vi "Power.vi"(8 "error in (no error)":errorcluster, 10 "Waveform in":waveform(dbl), 11 "RFID system in":refnum<class "RFID system.lvclass">) -> (0 "error out":errorcluster, 3 "RFID system out":refnum<class "RFID system.lvclass">, 5 "Waveform out":waveform(dbl))   [LabVIEW 2019, in "RFID system.lvclass"]
uses:
  RFID system.lvclass
  <vilib>/measure/madcrms.llb/Averaged DC-RMS for 1 Chan.vi
  <vilib>/measure/NI_MAPro.lvlib
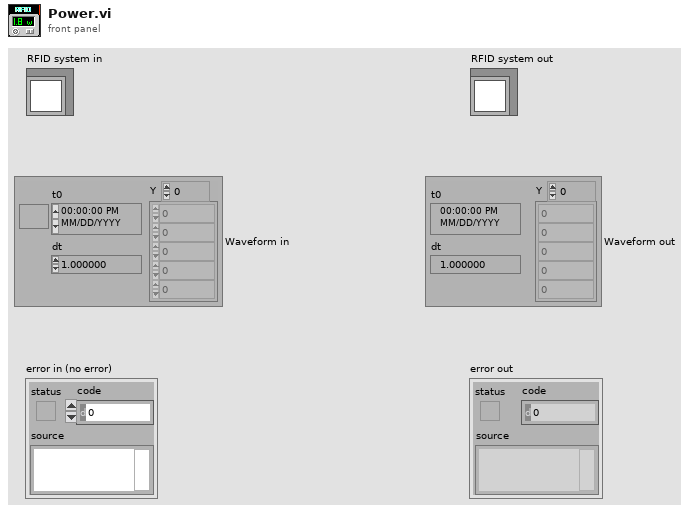
[diagram p1: front panel]
types:
  T1 = cluster{"window for DC":enum16{"Rectangular (none)", "Hanning", "Low side lobe"}, "output function":enum16{"DC only", "RMS only", "DC and RMS"}, "window for RMS":enum16{"Rectangular (none)", "Hanning", "Low side lobe"}, "exp. time constant":dbl, "Ignore input start time":bool}
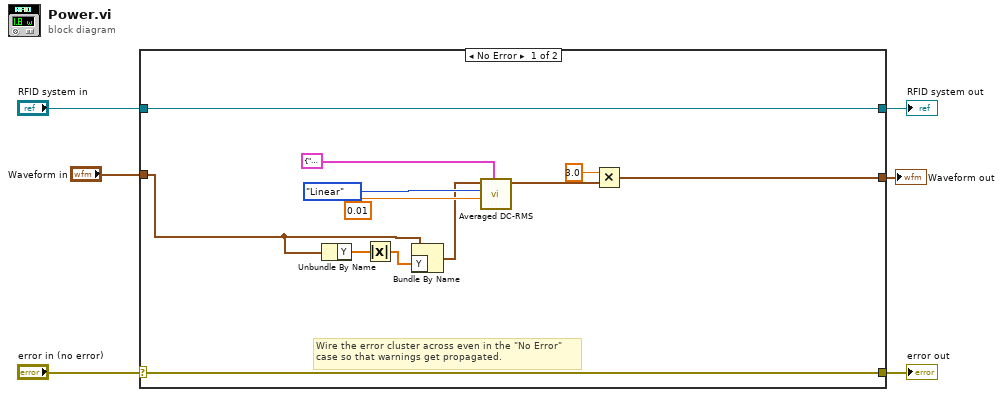
[diagram p0: block diagram]
diagram:
  n1 = case shown="No Error" "error in (no error)" {
    selector: "error in (no error)" -> [w17 w20]
    tunnel: [w17 w20] -> w5
    tunnel: [w18 w19] -> w3
    tunnel: "RFID system in" -> [w18 w19]
    tunnel: "Waveform in" -> [w9 _]
    tunnel: [w7 _] -> w1
    frame No Error {
      # "Wire the error cluster across even in the \"No Error\"\ncase so that warnings get propagated."
      n2 = Unbundle By Name(w9) -> ("Y"=w16:dbl[])
      n3 = Absolute Value(x=w16) -> (abs(x)=w15:dbl[])
      n4 = Bundle By Name(cluster=w9, "Y"=w15) -> (w8:waveform(dbl))
      n5 = call-poly <vilib>:"Averaged DC-RMS.vi"("averaging control"=T1 {"window for DC"=enum."Rectangular (none)", "output function"=enum."DC and RMS", "window for RMS"=enum."Rectangular (none)", "exp. time constant"=-1.0, "Ignore input start time"=FALSE}, "averaging time"=0.01, "averaging type"=enum16{"Linear", "Exponential"}."Linear", "signal in"=w8) -> ("DC value waveform"=w14:waveform(dbl))  [unwired: 3 in, 4 out]
      n6 = Multiply(x=3.0, y=w14) -> (x*y=w7:waveform(dbl))
    }
    frame Error {
    }
  }
  "error out" <- w5
  "RFID system out" <- w3
  "Waveform out" <- w1
